vi "Handle Command.vi"(8 "error in (no error)":errorcluster, 9 "Data":variant, 10 "Command":string, 11 "Instrument.Oxford1820 in":refnum<class "Instrument.Oxford1820.lvclass">) -> (0 "error out":errorcluster, 1 "Processed Data":variant, 2 "Command":string, 3 "Instrument.Oxford1820 out":refnum<class "Instrument.Oxford1820.lvclass">)   [LabVIEW 2019, in "Instrument.Oxford1820.lvclass"]
uses:
  Instrument.Oxford1820.lvclass
  Typedefs/Instrument.Oxford1820.protectedCommands-enum.ctl
  Typedefs/Instrument.Oxford1820.publicCommands-enum.ctl
  <userlib>/LevyLab/Instrument Framework/Instrument Types/Cryostat/Typedefs/getMagnet--cluster.ctl
  Instrument.Oxford1820.lvclass/Instrument.Oxford1820.ctl
  Typedefs/getLHeLevel--Cluster.ctl
  Typedefs/getLN2Level--Cluster.ctl
  Typedefs/PrivateEvents--Instrument.Oxford1820.setMagnet.ctl
  <userlib>/LevyLab/Instrument Framework/Instrument Types/Cryostat/Typedefs/Magnet Axis--Enum.ctl
  <userlib>/LevyLab/Instrument Framework/Instrument Types/Cryostat/Typedefs/Magnet Mode--Enum.ctl
  <userlib>/LevyLab/Instrument Framework/Instrument Types/Cryostat/Instrument.Cryostat.lvclass
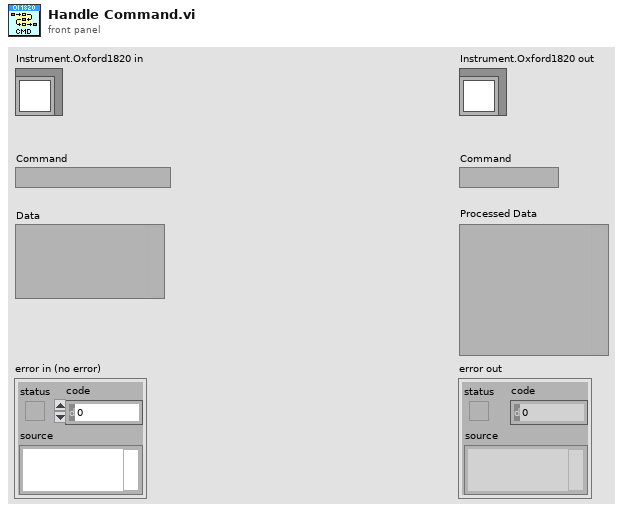
[diagram p1: front panel]
types:
  T1 = typedef "Instrument.Oxford1820.lvclass/Instrument.Oxford1820.publicCommands-enum.ctl" = enum16{"setMagnet", "getMagnet", "getMagnetTarget", "getLHeLevel", "getLN2level"}
  T2 = typedef "Instrument.Oxford1820.lvclass/Instrument.Oxford1820.protectedCommands-enum.ctl" = enum16{"Hold", "RampToSet", "RampToZero", "Clamp", "setTarget", "setSwitchHeat", "setLambda", "setFillMode", "setNeedleValve", "getStatus", "getTarget", "getSwitchHeat", "getPSUField", "setSequenceStatus"}
  T3 = typedef "Instrument.Cryostat.lvclass/getMagnet--cluster.ctl" = cluster{"field":dbl, "status":string, "finished":bool}
  T4 = typedef "Instrument.Oxford1820.lvclass/getLHeLevel--Cluster.ctl" = cluster{"LHeLevel":dbl}
  T5 = typedef "Instrument.Oxford1820.lvclass/getLN2Level--Cluster.ctl" = cluster{"LN2Level":dbl}
  T6 = typedef "Instrument.Oxford1820.lvclass/PrivateEvents--Instrument.Oxford1820.setMagnet.ctl" = cluster{"field":dbl, "rate":dbl, "axis":T7, "mode":T8}
  T7 = typedef "Instrument.Cryostat.lvclass/Magnet Axis--Enum.ctl" = enum16{"X", "Y", "Z"}
  T8 = typedef "Instrument.Cryostat.lvclass/Magnet Mode--Enum.ctl" = enum16{"Persistent", "Driven"}
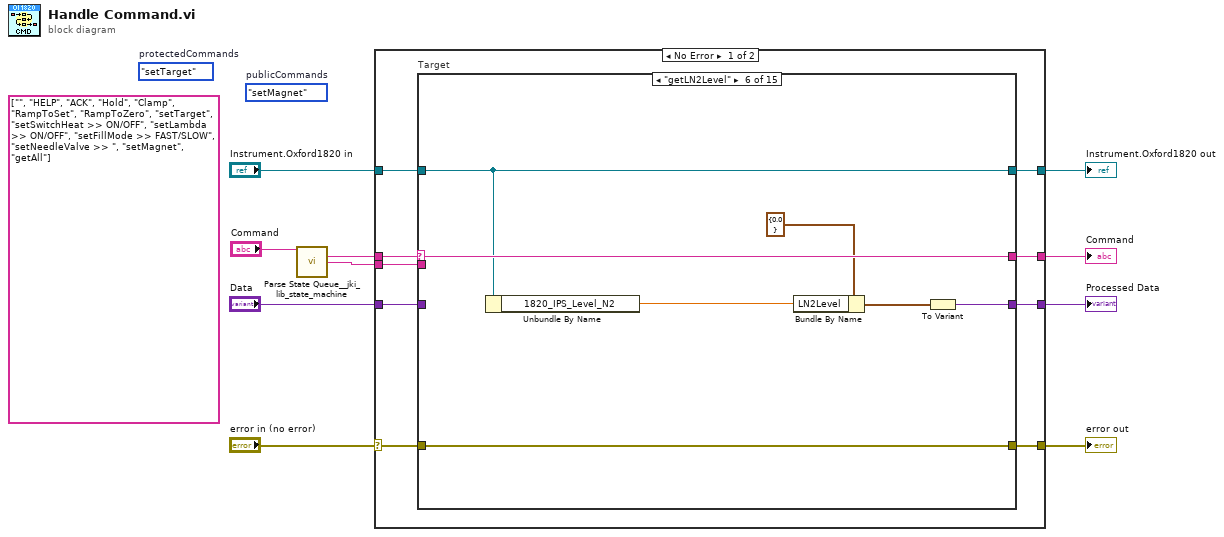
[diagram p0: block diagram]
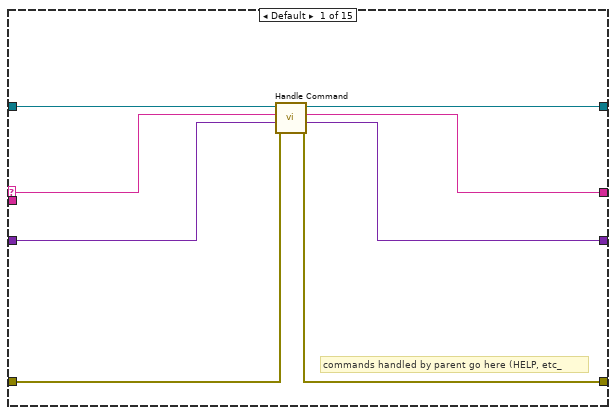
[diagram p2: hidden frame]
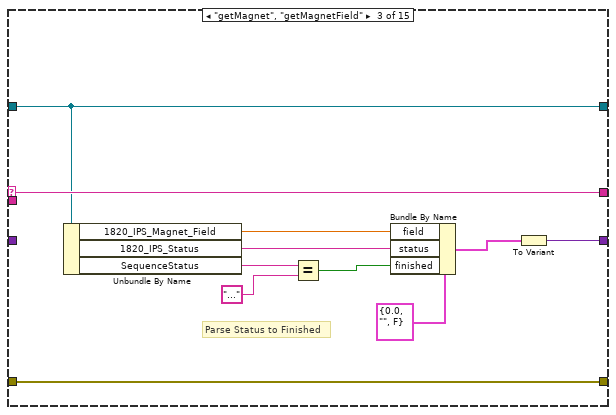
[diagram p4: hidden frame]
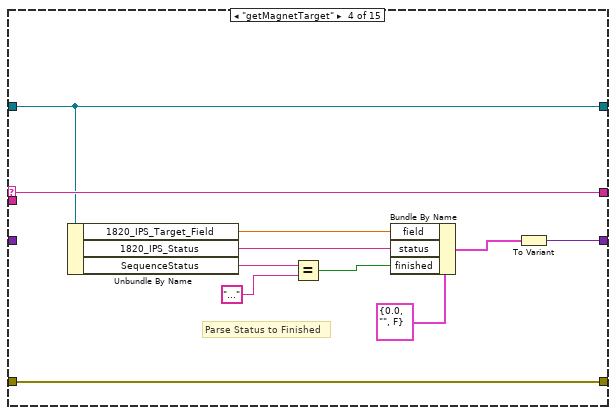
[diagram p5: hidden frame]
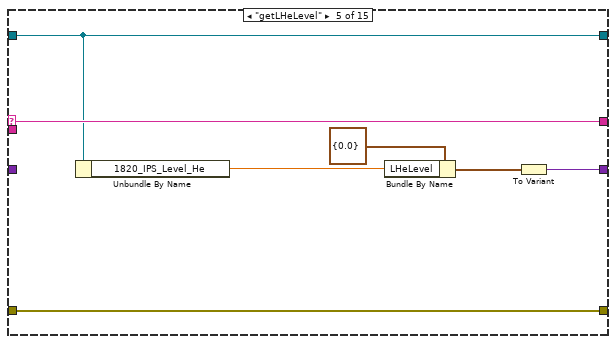
[diagram p6: hidden frame]
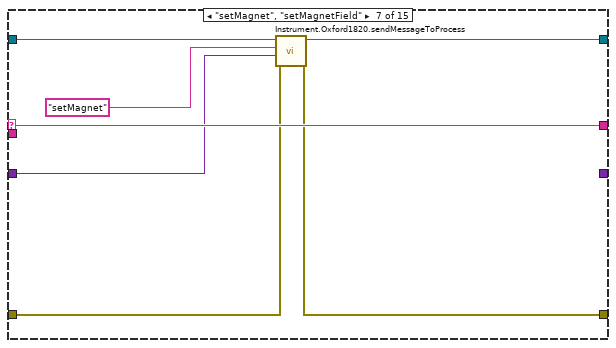
[diagram p7: hidden frame]
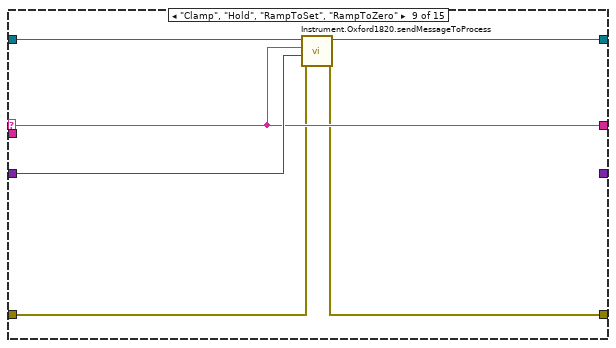
[diagram p9: hidden frame]
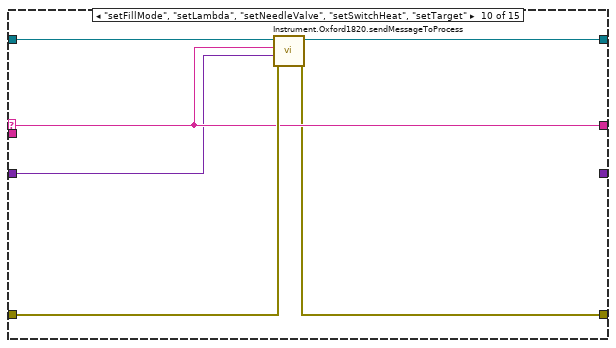
[diagram p10: hidden frame]
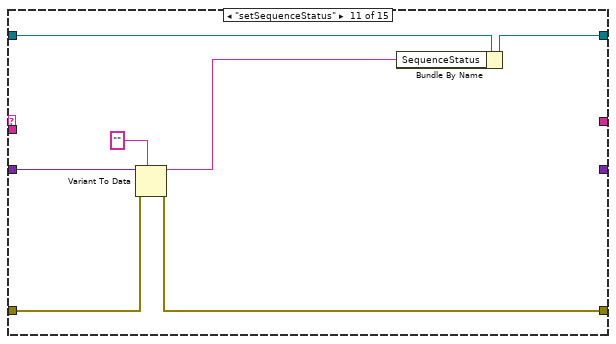
[diagram p11: hidden frame]
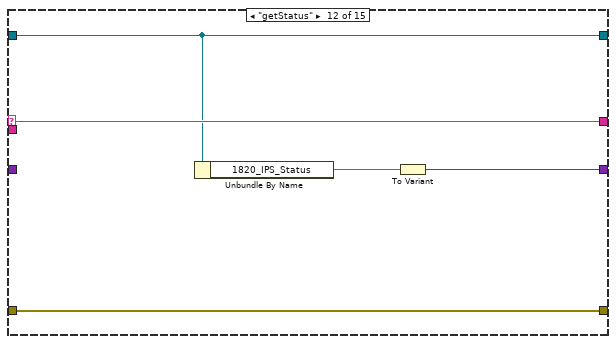
[diagram p12: hidden frame]
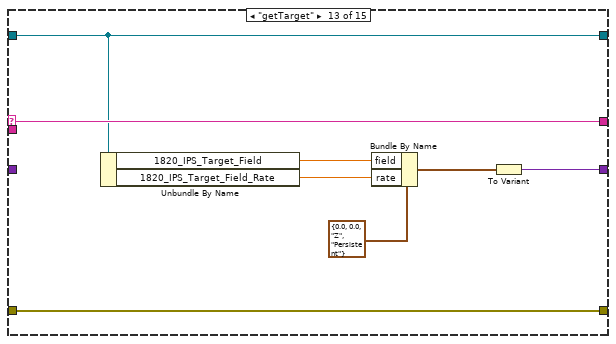
[diagram p13: hidden frame]
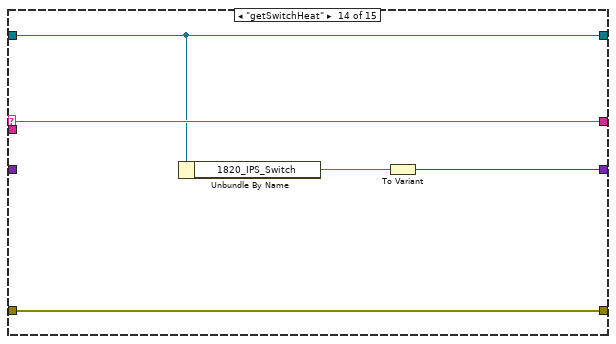
[diagram p14: hidden frame]
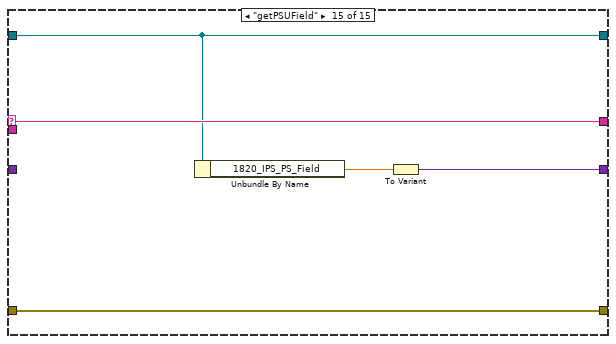
[diagram p15: hidden frame]
diagram:
  (unwired) Instrument.Oxford1820.publicCommands-enum."setMagnet"  # publicCommands
  (unwired) Instrument.Oxford1820.protectedCommands-enum."setTarget"  # protectedCommands
  (unwired) string[] ["", "HELP", "ACK", "Hold", "Clamp", "RampToSet", "RampToZero", "setTarget", "setSwitchHeat >> ON/OFF", "setLambda >> ON/OFF", "setFillMode >> FAST/SLOW", "setNeedleValve >> ", "setMagnet", "getAll"] ("Commands")
  n1 = call <vilib>:"Parse State Queue__jki_lib_state_machine.vi"("State Queue"="Command") -> ("Current State"=w4:string, "Arguments"=w3:string)  [unwired: 12 in, 1 out]
  n2 = case shown="No Error" "error in (no error)" {
    selector: "error in (no error)" -> [w11 w118]
    tunnel: [w15 w118] -> w10
    tunnel: [w19 w117] -> w9
    tunnel: [w18 _] -> w8
    tunnel: [w17 w119] -> w7
    tunnel: "Data" -> [w12 w117]
    tunnel: w4 -> [w13 _]
    tunnel: "Instrument.Oxford1820 in" -> [w16 w119]
    tunnel: w3 -> [w14 _]
    frame No Error {
      n3 = case "Target" shown="\"getLN2Level\"" w13 {
        selector: w13 -> [w22 _ w40 w51 w58 w65 w70 _ w78 w83 _ w98 w106 w111 w116]
        tunnel: [w20 _ w39 w50 w57 w64 _ _ _ _ _ w97 w105 w110 w115] -> w19
        tunnel: [w27 _ w40 w51 w58 w65 w70 _ w78 w83 _ w98 w106 w111 w116] -> w18
        tunnel: [w26 w29 w37 w48 w55 w62 w71 w74 w76 w84 w91 w94 w99 w107 w113] -> w17
        tunnel: w16 -> [w25 w29 w37 w48 w55 w62 w72 w74 w79 w85 w92 w94 w99 w107 w113]
        tunnel: w11 -> [w24 w28 w38 w49 w56 w63 w67 w73 w77 w86 w88 w96 w103 w109 w114]
        tunnel: [w23 w28 w38 w49 w56 w63 w69 w73 w75 w81 w87 w96 w103 w109 w114] -> w15
        tunnel: w14 -> [_ _ _ _ _ _ _ _ _ _ _ _ _ _ _]
        tunnel: w12 -> [w21 _ _ _ _ _ w68 _ w80 w82 w93 _ _ _ _]
        frame Default {
          # "commands handled by parent go here (HELP, etc_"
          n4 = call-parent "Handle Command.vi"("error in (no error)"=w24, "params in"=w21, "command"=w22, "Instrument in"=w25) -> ("error out"=w23:errorcluster, "processed data"=w20:variant, "command out"=w27:string, "Instrument out"=w26:refnum<class "Instrument.Oxford1820.lvclass">)  [unwired: 4 in]
        }
        frame "---public---" {
        }
        frame "getMagnet", "getMagnetField" {
          # "Parse Status to Finished"
          n5 = Unbundle By Name(w37) -> ("1820_IPS_Magnet_Field"=w36:dbl, "1820_IPS_Status"=w35:string, "SequenceStatus"=w32:string)
          n6 = Equal?(x=w32, y="...") -> (x = y?=w30:bool)
          n7 = Bundle By Name(cluster=T3 {"field"=0.0, "status"="", "finished"=FALSE} ("getMagnet"), "field"=w36, "status"=w35, "finished"=w30) -> (w34:T3)
          n8 = To Variant(anything=w34) -> (Variant=w39:variant)
        }
        frame "getMagnetTarget" {
          # "Parse Status to Finished"
          n9 = Unbundle By Name(w48) -> ("1820_IPS_Target_Field"=w47:dbl, "1820_IPS_Status"=w46:string, "SequenceStatus"=w43:string)
          n10 = Equal?(x=w43, y="...") -> (x = y?=w41:bool)
          n11 = Bundle By Name(cluster=T3 {"field"=0.0, "status"="", "finished"=FALSE} ("getMagnet"), "field"=w47, "status"=w46, "finished"=w41) -> (w45:T3)
          n12 = To Variant(anything=w45) -> (Variant=w50:variant)
        }
        frame "getLHeLevel" {
          n13 = Unbundle By Name(w55) -> ("1820_IPS_Level_He"=w53:dbl)
          n14 = Bundle By Name(cluster=T4 {"LHeLevel"=0.0} ("getHeLevel"), "LHeLevel"=w53) -> (w52:T4)
          n15 = To Variant(anything=w52) -> (Variant=w57:variant)
        }
        frame "getLN2Level" {
          n16 = Unbundle By Name(w62) -> ("1820_IPS_Level_N2"=w61:dbl)
          n17 = Bundle By Name(cluster=T5 {"LN2Level"=0.0} ("getN2Level"), "LN2Level"=w61) -> (w60:T5)
          n18 = To Variant(anything=w60) -> (Variant=w64:variant)
        }
        frame "setMagnet", "setMagnetField" {
          n19 = call "Instrument.Oxford1820.sendMessageToProcess.vi"("error in (no error)"=w67, "Data"=w68, "Command"="setMagnet", "Instrument.Oxford1820"=w72) -> ("error out"=w69:errorcluster, "Instrument.Oxford1820 out"=w71:refnum<class "Instrument.Oxford1820.lvclass">)  [unwired: 6 in]
        }
        frame "---protected---" {
        }
        frame "Clamp", "Hold", "RampToSet", "RampToZero" {
          n20 = call "Instrument.Oxford1820.sendMessageToProcess.vi"("error in (no error)"=w77, "Data"=w80, "Command"=w78, "Instrument.Oxford1820"=w79) -> ("error out"=w75:errorcluster, "Instrument.Oxford1820 out"=w76:refnum<class "Instrument.Oxford1820.lvclass">)  [unwired: 6 in]
        }
        frame "setFillMode", "setLambda", "setNeedleValve", "setSwitchHeat", "setTarget" {
          n21 = call "Instrument.Oxford1820.sendMessageToProcess.vi"("error in (no error)"=w86, "Data"=w82, "Command"=w83, "Instrument.Oxford1820"=w85) -> ("error out"=w81:errorcluster, "Instrument.Oxford1820 out"=w84:refnum<class "Instrument.Oxford1820.lvclass">)  [unwired: 6 in]
        }
        frame "setSequenceStatus" {
          n22 = Variant To Data(error in=w88, type="", Variant=w93) -> (data=w90:string, error out=w87:errorcluster)
          n23 = Bundle By Name(cluster=w92, "SequenceStatus"=w90) -> (w91:refnum<class "Instrument.Oxford1820.lvclass">)
        }
        frame "getStatus" {
          n24 = Unbundle By Name(w94) -> ("1820_IPS_Status"=w95:string)
          n25 = To Variant(anything=w95) -> (Variant=w97:variant)
        }
        frame "getTarget" {
          n26 = Unbundle By Name(w99) -> ("1820_IPS_Target_Field"=w101:dbl, "1820_IPS_Target_Field_Rate"=w100:dbl)
          n27 = Bundle By Name(cluster=T6 {"field"=0.0, "rate"=0.0, "axis"=enum."Z", "mode"=enum."Persistent"} ("Set Magnet Field"), "field"=w101, "rate"=w100) -> (w104:T6)
          n28 = To Variant(anything=w104) -> (Variant=w105:variant)
        }
        frame "getSwitchHeat" {
          n29 = Unbundle By Name(w107) -> ("1820_IPS_Switch"=w108:string)
          n30 = To Variant(anything=w108) -> (Variant=w110:variant)
        }
        frame "getPSUField" {
          n31 = Unbundle By Name(w113) -> ("1820_IPS_PS_Field"=w112:dbl)
          n32 = To Variant(anything=w112) -> (Variant=w115:variant)
        }
      }
    }
    frame Error {
    }
  }
  "error out" <- w10
  "Instrument.Oxford1820 out" <- w7
  "Processed Data" <- w9
  "Command" <- w8
